vi "Generate Event.vi"(4 "Error In":errorcluster, 5 "Response Notifier":string, 6 "Sample Period":i32, 7 "Source Name":string) -> (0 "Error Out":errorcluster)   [LabVIEW 2020, in "Set Acquisition Rate.lvlib"]
uses:
  Set Acquisition Rate.lvlib
  typedefs/Event Data.ctl
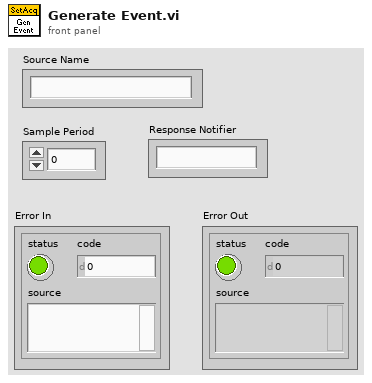
[diagram p1: front panel]
types:
  T1 = typedef "Set Acquisition Rate.lvlib/Event Data.ctl" = cluster{"Source Name":string, "Sample Period":i32, "Response Notifier":string}
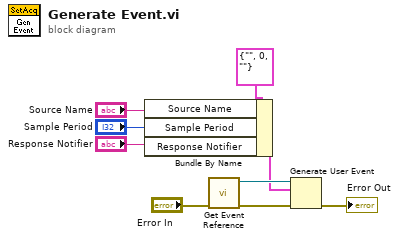
[diagram p0: block diagram]
diagram:
  n1 = Bundle By Name(cluster=T1 {"Source Name"="", "Sample Period"=0, "Response Notifier"=""} ("event data"), "Source Name"="Source Name", "Sample Period"="Sample Period", "Response Notifier"="Response Notifier") -> (w4:T1)
  n2 = call "Get Event Reference.vi"("error in (no error)"="Error In") -> ("error out"=w8:errorcluster, "Set Acquisition Rate"=w7:refnum<user-event>)  [unwired: 5 in]
  n3 = Generate User Event(user event=w7, event data cluster=w4, error in=w8) -> (error out=→"Error Out":errorcluster)  [unwired: 1 in, 1 out]
